vi "Get Valid Properties.vi"(8 "error in (no error)":errorcluster, 11 "File in":refnum<class "File.lvclass">) -> (0 "error out":errorcluster, 2 "Properties":string[](array[string]), 3 "File out":refnum<class "File.lvclass">)   [LabVIEW 2020, in "File.lvclass"]
uses:
  File.lvclass
  File.lvclass/File.ctl
  <vilib>/regexp/Match Regular Expression.xnode
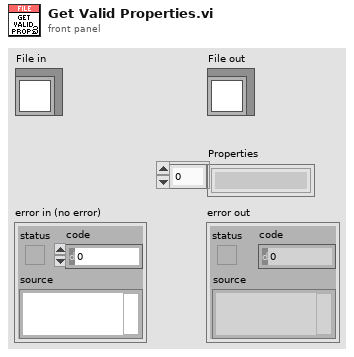
[diagram p1: front panel]
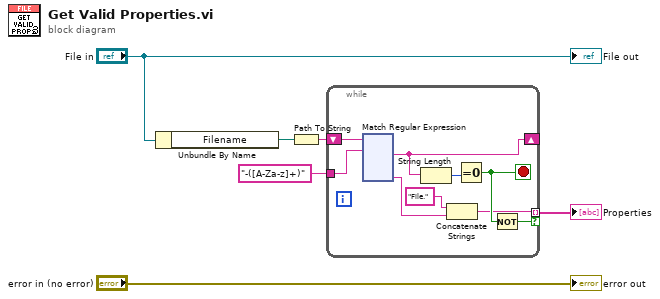
[diagram p0: block diagram]
diagram:
  n1 = Unbundle By Name("File in") -> ("Filename"=w1:path)
  n2 = Path To String(path=w1) -> (string=w5:string)
  n3 = while {
    tunnel: "-([A-Za-z]+)" ("regular expression") -> [w14]
    tunnel: [w9] -> w4 mode=indexing if=w11
    shift-right: [w12] -> _
    shift-left: w5 -> [w15]
    stop <- w10 stop-if-true
    n4 = xnode "Match Regular Expression"("input string"=w15, "regular expression"=w14) -> ("after match"=w12:string, "submatch 1"=w8:string)  [unwired: 4 in, 4 out]
    n5 = String Length(string=w12) -> (length=w13:i32)
    n6 = Concatenate Strings("File." ("string"), w8) -> (w9:string)
    n7 = Equal To 0?(x=w13) -> (x = 0?=w10:bool)
    n8 = Not(x=w10) -> (.not. x?=w11:bool)
  }
  "Properties" <- w4
  "error out" <- "error in (no error)"
  "File out" <- "File in"
